vi "Append Timeseries.vi"(7 "Duration":dbl[unit]=3333.0, 9 "Reset":bool, 10 "In New":T1, 11 "In Old":T1) -> (3 "Appended":T1)   [LabVIEW 2010]
panel:
  out "N samples":u32=3333
  out "Duration samples":u32=3333
  out "Sample time":dbl[unit]=3333.0
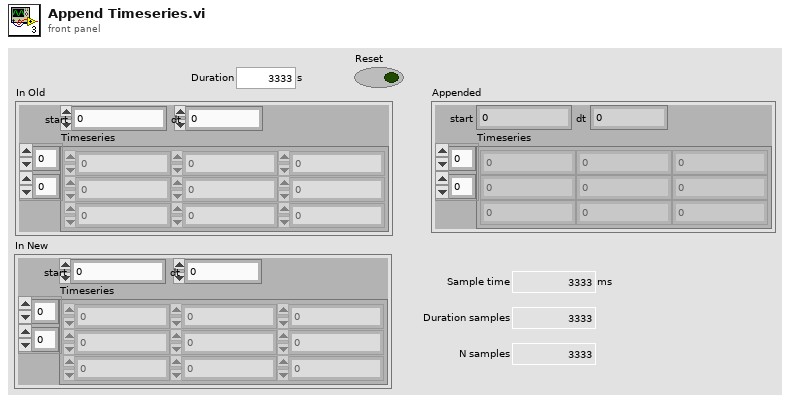
[diagram p1: front panel]
types:
  T1 = cluster{"start":dbl, "dt":dbl, "Timeseries":dbl[][]}
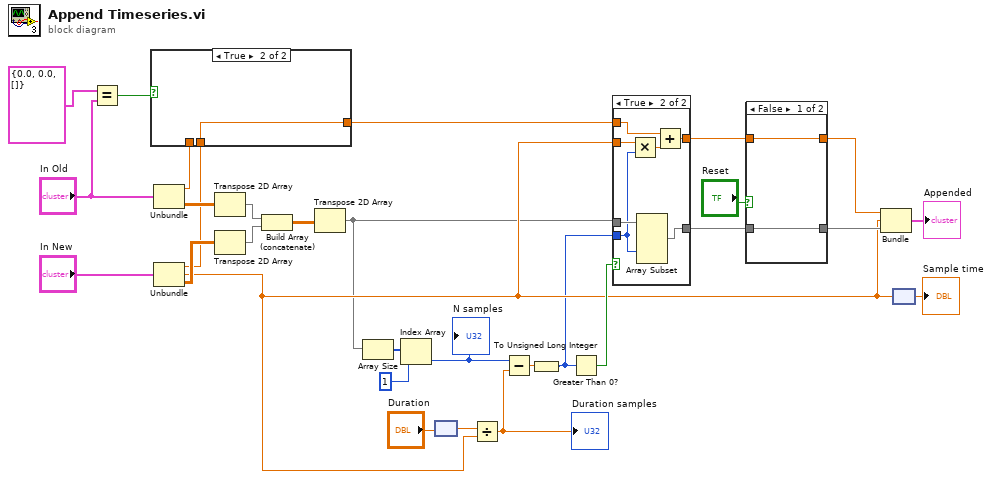
[diagram p0: block diagram]
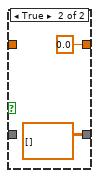
[diagram p3: hidden frame]
diagram:
  n1 = Equal?(x=cluster{dbl, dbl, dbl[][]} {0.0, 0.0, []} ("Waveform Timeseries"), y="In Old") -> (x = y?=w6:bool)
  n2 = Unbundle("In Old") -> ("start"=w3:dbl, "Timeseries"=w20:dbl[][])  [unwired: 1 out]
  n3 = Unbundle("In New") -> ("start"=w4:dbl, "dt"=w13:dbl, "Timeseries"=w18:dbl[][])
  n4 = case shown="True" w6 {
    tunnel: [w31 w32] -> w5
    tunnel: w4 -> [_ w32]
    tunnel: w3 -> [w31 _]
    frame False {
    }
    frame True {
    }
  }
  n5 = Transpose 2D Array(2D array=w20) -> (transposed array=w19:dbl[][])
  n6 = Transpose 2D Array(2D array=w18) -> (transposed array=w17:dbl[][])
  n7 = Build Array (concatenate)(w19, w17) -> (w16:dbl[][])
  n8 = Transpose 2D Array(2D array=w16) -> (transposed array=w9:dbl[][])
  n9 = Array Size(array=w9) -> (size(s)=w25:i32[])
  n10 = Index Array(array=w25, index=1) -> (element=w10:i32)
  "N samples" <- w10
  n11 = node("Duration") -> (w21:dbl)
  n12 = Divide(x=w21, y=w13) -> (x/y=w11:dbl)
  "Duration samples" <- w11
  n13 = Subtract(x=w10, y=w11) -> (x-y=w2:dbl)
  n14 = To Unsigned Long Integer(number=w2) -> (unsigned 32bit integer=w1:u32)
  n15 = Greater Than 0?(x=w1) -> (x > 0?=w22:bool)
  n16 = case shown="True" w22 {
    tunnel: [w34 w40] -> w29
    tunnel: w9 -> [w34 w41]
    tunnel: w1 -> [_ w35]
    tunnel: w13 -> [_ w39]
    tunnel: w5 -> [w33 w38]
    tunnel: [w33 w36] -> w15
    frame False {
    }
    frame True {
      n17 = Multiply(x=w39, y=w35) -> (x*y=w37:dbl)
      n18 = Array Subset(array=w41, index (col)=w35) -> (w40:dbl[][])  [unwired: 3 in]
      n19 = Add(x=w38, y=w37) -> (x+y=w36:dbl)
    }
  }
  n20 = case shown="False" "Reset" {
    tunnel: w29 -> [w43 _]
    tunnel: [w43 dbl[][] []] -> w26
    tunnel: w15 -> [w42 _]
    tunnel: [w42 0.0] -> w14
    frame False {
    }
    frame True {
    }
  }
  n21 = Bundle("start"=w14, "dt"=w13, w26) -> (→"Appended":cluster{"start":dbl, "dt":dbl, dbl[][]})  [unwired: 1 in]
  n22 = node(w13) -> (→"Sample time":dbl[unit])
